vi "Defaults.vi"(8 "error in (no error)":errorcluster, 11 "MB Slave in":refnum<class "Battery Pack.lvclass">) -> (0 "error out":errorcluster, 3 "MB Slave out":refnum<class "Battery Pack.lvclass">)   [LabVIEW 2021, in "Battery Pack.lvclass"]
uses:
  Battery Pack.lvclass
  C:/Program Files (x86)/National Instruments/LabVIEW 2021/user.lib/S2 Labs/Module Framework/Modules/Base/Module.lvclass
  C:/Program Files (x86)/National Instruments/LabVIEW 2021/user.lib/S2 Labs/Module Framework/Modules/Modbus/Modbus Slave Base/Modbus Slave Base.lvclass
  <userlib>/S2 Labs/Modbus Toolkit/TypeDefs/MB Element.ctl
  <userlib>/S2 Labs/Modbus Toolkit/TypeDefs/Endianness Type.ctl
  <userlib>/S2 Labs/Modbus Toolkit/TypeDefs/Access Type.ctl
  <userlib>/S2 Labs/Module Framework/Modules/Base/Module.lvclass/Module.ctl
  <userlib>/S2 Labs/Module Framework/Modules/Modbus/Modbus Slave Base/Modbus Slave Base.lvclass/Modbus Slave Base.ctl
  <userlib>/S2 Labs/Module Framework/Modules/Base/Read Name.vi
  <userlib>/S2 Labs/Module Framework/Modules/Modbus/Modbus Slave Base/Write MB Map.vi
  <userlib>/S2 Labs/Module Framework/Modules/Base/Write Timeout (ms).vi
  MB Slave Simulator Base/MB Slave Simulator Base.lvclass
  <userlib>/S2 Labs/Modbus Toolkit/S2L Modbus API.lvclass
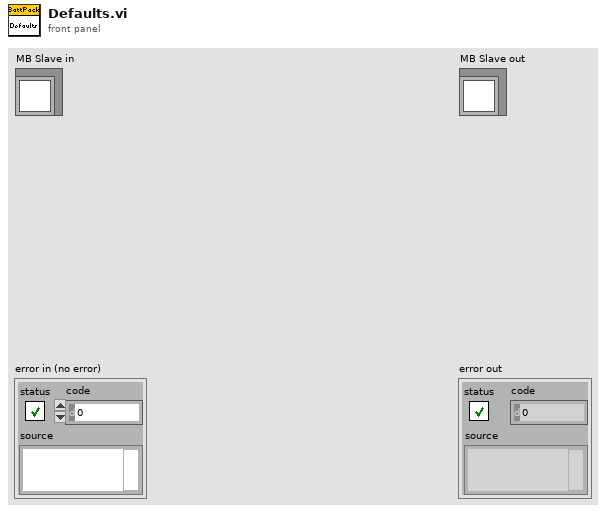
[diagram p1: front panel]
types:
  T1 = typedef "S2L Modbus API.lvclass/MB Element.ctl" = cluster{"Label":string, "Prefix":u8, "Address":u16, "Datatype":string, "Register Count":u8, "Multiplier":dbl, "Offset":dbl, "Unit":string, "Endianness":T2, "Access":T3, "LUT":string[], "Poll Rate(ms)":u16, "Mapping":cluster{"Module":string, "Channel":string}}
  T2 = typedef "Endianness Type.ctl" = enum16{"Big-Endian", "Little-Endian", "Big-Endian Byte Swap", "Little-Endian Byte Swap"}
  T3 = typedef "S2L Modbus API.lvclass/Access Type.ctl" = enum16{"R/W", "R", "W"}
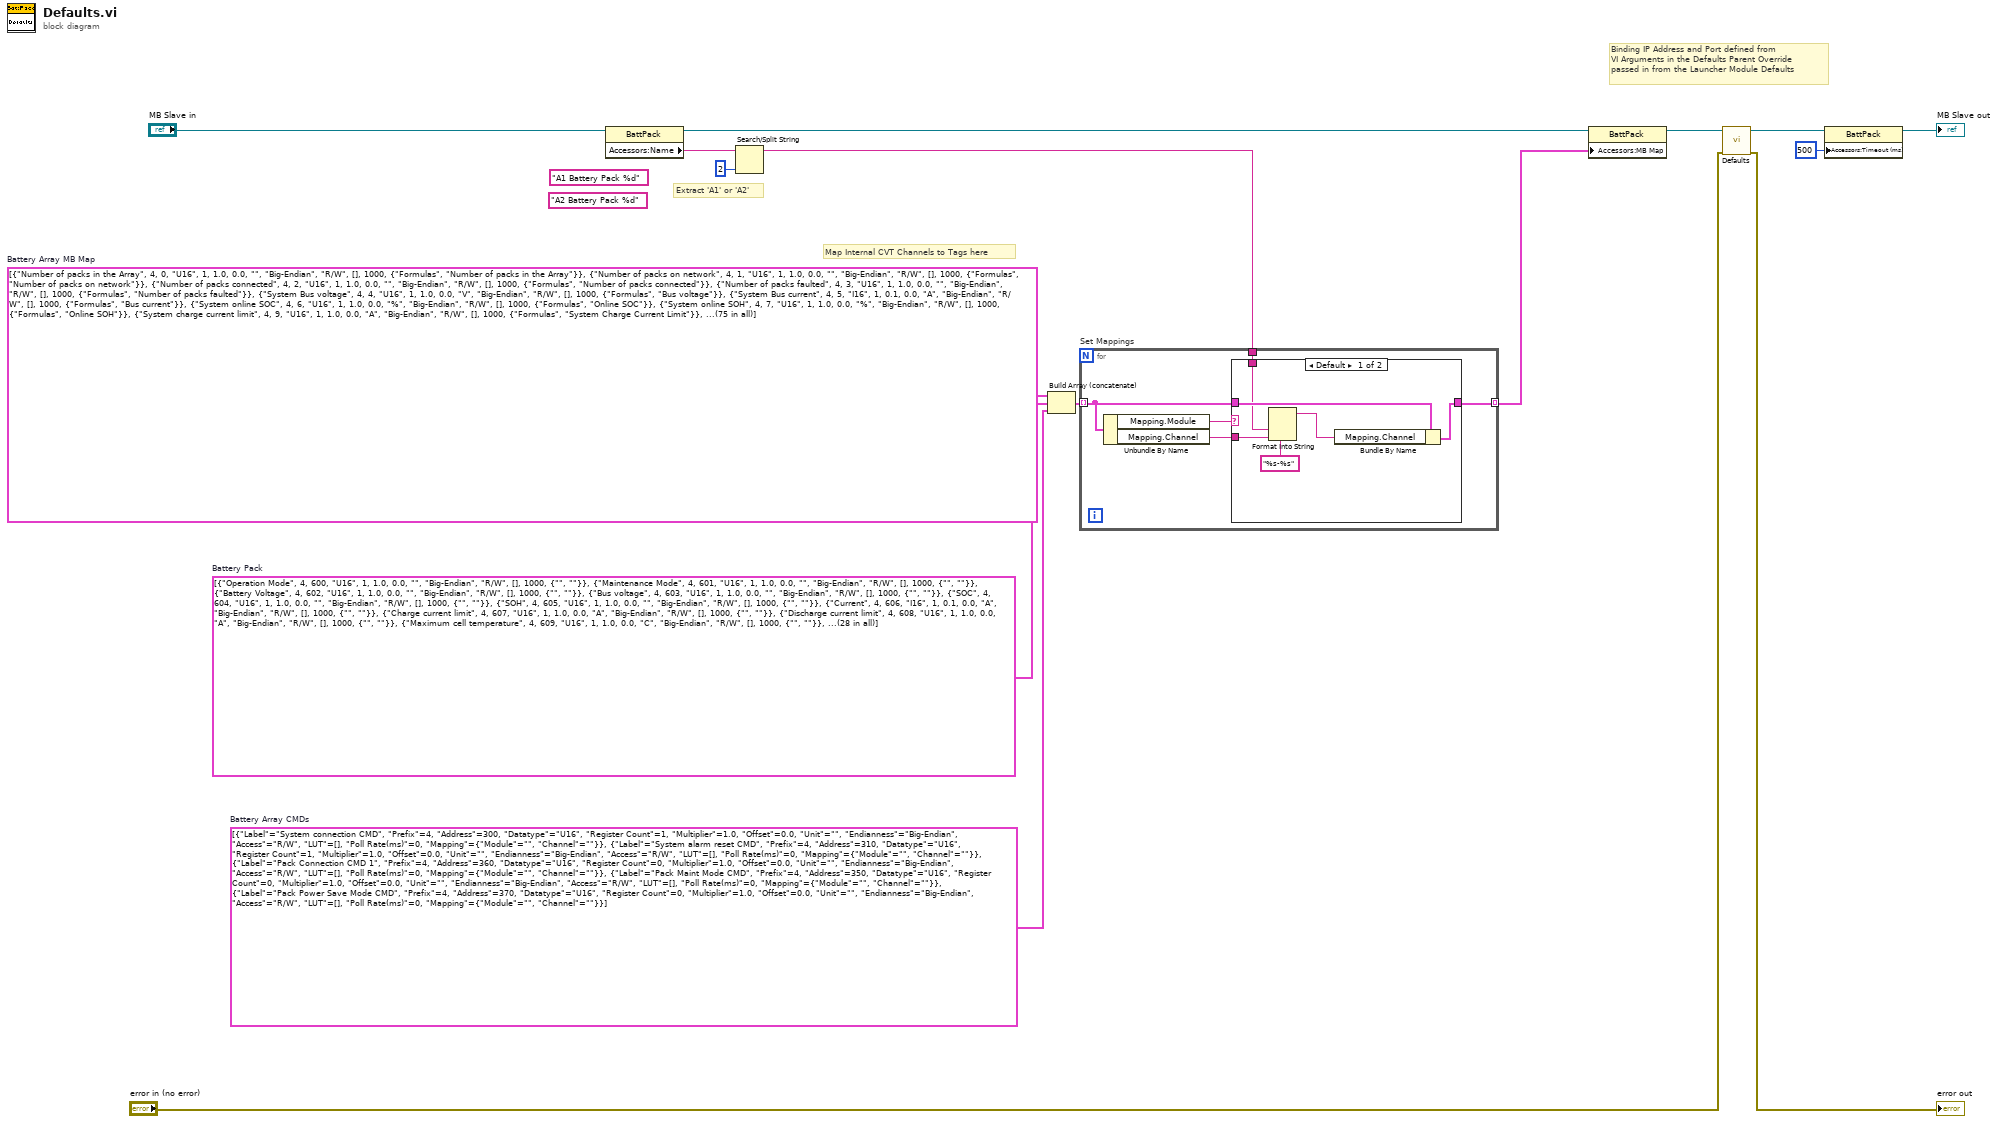
[diagram p0: block diagram]
diagram:
  (unwired) "A2 Battery Pack %d"
  (unwired) "A1 Battery Pack %d"
  w11 = T1[] [{"Label"="System connection CMD", "Prefix"=4, "Address"=300, "Datatype"="U16", "Register Count"=1, "Multiplier"=1.0, "Offset"=0.0, "Unit"="", "Endianness"=enum."Big-Endian", "Access"=enum."R/W", "LUT"=[], "Poll Rate(ms)"=0, "Mapping"={"Module"="", "Channel"=""}}, {"Label"="System alarm reset CMD", "Prefix"=4, "Address"=310, "Datatype"="U16", "Register Count"=1, "Multiplier"=1.0, "Offset"=0.0, "Unit"="", "Endianness"=enum."Big-Endian", "Access"=enum."R/W", "LUT"=[], "Poll Rate(ms)"=0, "Mapping"={"Module"="", "Channel"=""}}, {"Label"="Pack Connection CMD 1", "Prefix"=4, "Address"=360, "Datatype"="U16", "Register Count"=0, "Multiplier"=1.0, "Offset"=0.0, "Unit"="", "Endianness"=enum."Big-Endian", "Access"=enum."R/W", "LUT"=[], "Poll Rate(ms)"=0, "Mapping"={"Module"="", "Channel"=""}}, {"Label"="Pack Maint Mode CMD", "Prefix"=4, "Address"=350, "Datatype"="U16", "Register Count"=0, "Multiplier"=1.0, "Offset"=0.0, "Unit"="", "Endianness"=enum."Big-Endian", "Access"=enum."R/W", "LUT"=[], "Poll Rate(ms)"=0, "Mapping"={"Module"="", "Channel"=""}}, {"Label"="Pack Power Save Mode CMD", "Prefix"=4, "Address"=370, "Datatype"="U16", "Register Count"=0, "Multiplier"=1.0, "Offset"=0.0, "Unit"="", "Endianness"=enum."Big-Endian", "Access"=enum."R/W", "LUT"=[], "Poll Rate(ms)"=0, "Mapping"={"Module"="", "Channel"=""}}]  # Battery Array CMDs
  w13 = T1[] [{"Label"="Number of packs in the Array", "Prefix"=4, "Address"=0, "Datatype"="U16", "Register Count"=1, "Multiplier"=1.0, "Offset"=0.0, "Unit"="", "Endianness"=enum."Big-Endian", "Access"=enum."R/W", "LUT"=[], "Poll Rate(ms)"=1000, "Mapping"={"Module"="Formulas", "Channel"="Number of packs in the Array"}}, {"Label"="Number of packs on network", "Prefix"=4, "Address"=1, "Datatype"="U16", "Register Count"=1, "Multiplier"=1.0, "Offset"=0.0, "Unit"="", "Endianness"=enum."Big-Endian", "Access"=enum."R/W", "LUT"=[], "Poll Rate(ms)"=1000, "Mapping"={"Module"="Formulas", "Channel"="Number of packs on network"}}, {"Label"="Number of packs connected", "Prefix"=4, "Address"=2, "Datatype"="U16", "Register Count"=1, "Multiplier"=1.0, "Offset"=0.0, "Unit"="", "Endianness"=enum."Big-Endian", "Access"=enum."R/W", "LUT"=[], "Poll Rate(ms)"=1000, "Mapping"={"Module"="Formulas", "Channel"="Number of packs connected"}}, {"Label"="Number of packs faulted", "Prefix"=4, "Address"=3, "Datatype"="U16", "Register Count"=1, "Multiplier"=1.0, "Offset"=0.0, "Unit"="", "Endianness"=enum."Big-Endian", "Access"=enum."R/W", "LUT"=[], "Poll Rate(ms)"=1000, "Mapping"={"Module"="Formulas", "Channel"="Number of packs faulted"}}, {"Label"="System Bus voltage", "Prefix"=4, "Address"=4, "Datatype"="U16", "Register Count"=1, "Multiplier"=1.0, "Offset"=0.0, "Unit"="V", "Endianness"=enum."Big-Endian", "Access"=enum."R/W", "LUT"=[], "Poll Rate(ms)"=1000, "Mapping"={"Module"="Formulas", "Channel"="Bus voltage"}}, {"Label"="System Bus current", "Prefix"=4, "Address"=5, "Datatype"="I16", "Register Count"=1, "Multiplier"=0.1, "Offset"=0.0, "Unit"="A", "Endianness"=enum."Big-Endian", "Access"=enum."R/W", "LUT"=[], "Poll Rate(ms)"=1000, "Mapping"={"Module"="Formulas", "Channel"="Bus current"}}, {"Label"="System online SOC", "Prefix"=4, "Address"=6, "Datatype"="U16", "Register Count"=1, "Multiplier"=1.0, "Offset"=0.0, "Unit"="%", "Endianness"=enum."Big-Endian", "Access"=enum."R/W", "LUT"=[], "Poll Rate(ms)"=1000, "Mapping"={"Module"="Formulas", "Channel"="Online SOC"}}, {"Label"="System online SOH", "Prefix"=4, "Address"=7, "Datatype"="U16", "Register Count"=1, "Multiplier"=1.0, "Offset"=0.0, "Unit"="%", "Endianness"=enum."Big-Endian", "Access"=enum."R/W", "LUT"=[], "Poll Rate(ms)"=1000, "Mapping"={"Module"="Formulas", "Channel"="Online SOH"}}, {"Label"="System charge current limit", "Prefix"=4, "Address"=9, "Datatype"="U16", "Register Count"=1, "Multiplier"=1.0, "Offset"=0.0, "Unit"="A", "Endianness"=enum."Big-Endian", "Access"=enum."R/W", "LUT"=[], "Poll Rate(ms)"=1000, "Mapping"={"Module"="Formulas", "Channel"="System Charge Current Limit"}}, {"Label"="System discharge current limit", "Prefix"=4, "Address"=10, "Datatype"="U16", "Register Count"=1, "Multiplier"=1.0, "Offset"=0.0, "Unit"="A", "Endianness"=enum."Big-Endian", "Access"=enum."R/W", "LUT"=[], "Poll Rate(ms)"=1000, "Mapping"={"Module"="Formulas", "Channel"="System Discharge Current Limit"}}, {"Label"="System Maximum cell temperature", "Prefix"=4, "Address"=11, "Datatype"="I16", "Register Count"=1, "Multiplier"=1.0, "Offset"=0.0, "Unit"="C", "Endianness"=enum."Big-Endian", "Access"=enum."R/W", "LUT"=[], "Poll Rate(ms)"=1000, "Mapping"={"Module"="Formulas", "Channel"="Max Online Cell Temp"}}, {"Label"="System Minimum cell temperature", "Prefix"=4, "Address"=12, "Datatype"="I16", "Register Count"=1, "Multiplier"=1.0, "Offset"=0.0, "Unit"="C", "Endianness"=enum."Big-Endian", "Access"=enum."R/W", "LUT"=[], "Poll Rate(ms)"=1000, "Mapping"={"Module"="", "Channel"=""}}, {"Label"="System Maximum cell voltage", "Prefix"=4, "Address"=13, "Datatype"="U16", "Register Count"=1, "Multiplier"=1.0, "Offset"=0.0, "Unit"="mV", "Endianness"=enum."Big-Endian", "Access"=enum."R/W", "LUT"=[], "Poll Rate(ms)"=1000, "Mapping"={"Module"="", "Channel"=""}}, {"Label"="System Minimum cell voltage", "Prefix"=4, "Address"=14, "Datatype"="U16", "Register Count"=1, "Multiplier"=1.0, "Offset"=0.0, "Unit"="mV", "Endianness"=enum."Big-Endian", "Access"=enum."R/W", "LUT"=[], "Poll Rate(ms)"=1000, "Mapping"={"Module"="", "Channel"=""}}, {"Label"="System Maximum unconnected pack voltage", "Prefix"=4, "Address"=15, "Datatype"="U16", "Register Count"=1, "Multiplier"=1.0, "Offset"=0.0, "Unit"="V", "Endianness"=enum."Big-Endian", "Access"=enum."R/W", "LUT"=[], "Poll Rate(ms)"=1000, "Mapping"={"Module"="", "Channel"=""}}, {"Label"="System Minimum unconnected pack voltage", "Prefix"=4, "Address"=16, "Datatype"="U16", "Register Count"=1, "Multiplier"=1.0, "Offset"=0.0, "Unit"="V", "Endianness"=enum."Big-Endian", "Access"=enum."R/W", "LUT"=[], "Poll Rate(ms)"=1000, "Mapping"={"Module"="", "Channel"=""}}, {"Label"="Pack heartbeat", "Prefix"=4, "Address"=17, "Datatype"="U32", "Register Count"=1, "Multiplier"=1.0, "Offset"=0.0, "Unit"="", "Endianness"=enum."Little-Endian", "Access"=enum."R/W", "LUT"=[], "Poll Rate(ms)"=1000, "Mapping"={"Module"="", "Channel"=""}}, {"Label"="Service state", "Prefix"=4, "Address"=19, "Datatype"="U16", "Register Count"=1, "Multiplier"=1.0, "Offset"=0.0, "Unit"="", "Endianness"=enum."Big-Endian", "Access"=enum."R/W", "LUT"=[], "Poll Rate(ms)"=1000, "Mapping"={"Module"="", "Channel"=""}}, {"Label"="Bus current unscaled", "Prefix"=4, "Address"=20, "Datatype"="I16", "Register Count"=1, "Multiplier"=1.0, "Offset"=0.0, "Unit"="A", "Endianness"=enum."Big-Endian", "Access"=enum."R/W", "LUT"=[], "Poll Rate(ms)"=1000, "Mapping"={"Module"="", "Channel"=""}}, {"Label"="Minimum pack SOC", "Prefix"=4, "Address"=21, "Datatype"="U16", "Register Count"=1, "Multiplier"=1.0, "Offset"=0.0, "Unit"="%", "Endianness"=enum."Big-Endian", "Access"=enum."R/W", "LUT"=[], "Poll Rate(ms)"=0, "Mapping"={"Module"="", "Channel"=""}}, {"Label"="Average pack SOC", "Prefix"=4, "Address"=22, "Datatype"="U16", "Register Count"=1, "Multiplier"=1.0, "Offset"=0.0, "Unit"="%", "Endianness"=enum."Big-Endian", "Access"=enum."R/W", "LUT"=[], "Poll Rate(ms)"=0, "Mapping"={"Module"="", "Channel"=""}}, {"Label"="Maximum pack SOC", "Prefix"=4, "Address"=23, "Datatype"="U16", "Register Count"=1, "Multiplier"=1.0, "Offset"=0.0, "Unit"="%", "Endianness"=enum."Big-Endian", "Access"=enum."R/W", "LUT"=[], "Poll Rate(ms)"=0, "Mapping"={"Module"="", "Channel"=""}}, {"Label"="Average connected cell SOC", "Prefix"=4, "Address"=24, "Datatype"="U16", "Register Count"=1, "Multiplier"=1.0, "Offset"=0.0, "Unit"="%", "Endianness"=enum."Big-Endian", "Access"=enum."R/W", "LUT"=[], "Poll Rate(ms)"=0, "Mapping"={"Module"="", "Channel"=""}}, {"Label"="Maximum connected cell SOC", "Prefix"=4, "Address"=25, "Datatype"="U16", "Register Count"=1, "Multiplier"=1.0, "Offset"=0.0, "Unit"="%", "Endianness"=enum."Big-Endian", "Access"=enum."R/W", "LUT"=[], "Poll Rate(ms)"=0, "Mapping"={"Module"="", "Channel"=""}}, {"Label"="Pack 1 operation mode", "Prefix"=4, "Address"=50, "Datatype"="U16", "Register Count"=1, "Multiplier"=1.0, "Offset"=0.0, "Unit"="", "Endianness"=enum."Big-Endian", "Access"=enum."R/W", "LUT"=[], "Poll Rate(ms)"=1000, "Mapping"={"Module"="Formulas", "Channel"="Pack 1 operation mode"}}, {"Label"="Pack 2 operation mode", "Prefix"=4, "Address"=51, "Datatype"="U16", "Register Count"=1, "Multiplier"=1.0, "Offset"=0.0, "Unit"="", "Endianness"=enum."Big-Endian", "Access"=enum."R/W", "LUT"=[], "Poll Rate(ms)"=1000, "Mapping"={"Module"="Formulas", "Channel"="Pack 2 operation mode"}}, {"Label"="Pack 3 operation mode", "Prefix"=4, "Address"=52, "Datatype"="U16", "Register Count"=1, "Multiplier"=1.0, "Offset"=0.0, "Unit"="", "Endianness"=enum."Big-Endian", "Access"=enum."R/W", "LUT"=[], "Poll Rate(ms)"=1000, "Mapping"={"Module"="Formulas", "Channel"="Pack 3 operation mode"}}, {"Label"="Pack 4 operation mode", "Prefix"=4, "Address"=53, "Datatype"="U16", "Register Count"=1, "Multiplier"=1.0, "Offset"=0.0, "Unit"="", "Endianness"=enum."Big-Endian", "Access"=enum."R/W", "LUT"=[], "Poll Rate(ms)"=1000, "Mapping"={"Module"="Formulas", "Channel"="Pack 4 operation mode"}}, {"Label"="Pack 5 operation mode", "Prefix"=4, "Address"=54, "Datatype"="U16", "Register Count"=1, "Multiplier"=1.0, "Offset"=0.0, "Unit"="", "Endianness"=enum."Big-Endian", "Access"=enum."R/W", "LUT"=[], "Poll Rate(ms)"=1000, "Mapping"={"Module"="Formulas", "Channel"="Pack 5 operation mode"}}, {"Label"="Pack 6 operation mode", "Prefix"=4, "Address"=55, "Datatype"="U16", "Register Count"=1, "Multiplier"=1.0, "Offset"=0.0, "Unit"="", "Endianness"=enum."Big-Endian", "Access"=enum."R/W", "LUT"=[], "Poll Rate(ms)"=1000, "Mapping"={"Module"="Formulas", "Channel"="Pack 6 operation mode"}}, {"Label"="Pack 1 maintenance status", "Prefix"=4, "Address"=66, "Datatype"="U16", "Register Count"=1, "Multiplier"=1.0, "Offset"=0.0, "Unit"="", "Endianness"=enum."Big-Endian", "Access"=enum."R/W", "LUT"=[], "Poll Rate(ms)"=1000, "Mapping"={"Module"="", "Channel"=""}}, {"Label"="Pack 2 maintenance status", "Prefix"=4, "Address"=67, "Datatype"="U16", "Register Count"=1, "Multiplier"=1.0, "Offset"=0.0, "Unit"="", "Endianness"=enum."Big-Endian", "Access"=enum."R/W", "LUT"=[], "Poll Rate(ms)"=1000, "Mapping"={"Module"="", "Channel"=""}}, {"Label"="Pack 3 maintenance status", "Prefix"=4, "Address"=68, "Datatype"="U16", "Register Count"=1, "Multiplier"=1.0, "Offset"=0.0, "Unit"="", "Endianness"=enum."Big-Endian", "Access"=enum."R/W", "LUT"=[], "Poll Rate(ms)"=1000, "Mapping"={"Module"="", "Channel"=""}}, {"Label"="Pack 4 maintenance status", "Prefix"=4, "Address"=69, "Datatype"="U16", "Register Count"=1, "Multiplier"=1.0, "Offset"=0.0, "Unit"="", "Endianness"=enum."Big-Endian", "Access"=enum."R/W", "LUT"=[], "Poll Rate(ms)"=1000, "Mapping"={"Module"="", "Channel"=""}}, {"Label"="Pack 5 maintenance status", "Prefix"=4, "Address"=70, "Datatype"="U16", "Register Count"=1, "Multiplier"=1.0, "Offset"=0.0, "Unit"="", "Endianness"=enum."Big-Endian", "Access"=enum."R/W", "LUT"=[], "Poll Rate(ms)"=1000, "Mapping"={"Module"="", "Channel"=""}}, {"Label"="Pack 6 maintenance status", "Prefix"=4, "Address"=71, "Datatype"="U16", "Register Count"=1, "Multiplier"=1.0, "Offset"=0.0, "Unit"="", "Endianness"=enum."Big-Endian", "Access"=enum."R/W", "LUT"=[], "Poll Rate(ms)"=1000, "Mapping"={"Module"="", "Channel"=""}}, {"Label"="Pack 1 pre-charge status", "Prefix"=4, "Address"=82, "Datatype"="U16", "Register Count"=1, "Multiplier"=1.0, "Offset"=0.0, "Unit"="", "Endianness"=enum."Big-Endian", "Access"=enum."R/W", "LUT"=[], "Poll Rate(ms)"=1000, "Mapping"={"Module"="", "Channel"=""}}, {"Label"="Pack 2 pre-charge status", "Prefix"=4, "Address"=83, "Datatype"="U16", "Register Count"=1, "Multiplier"=1.0, "Offset"=0.0, "Unit"="", "Endianness"=enum."Big-Endian", "Access"=enum."R/W", "LUT"=[], "Poll Rate(ms)"=1000, "Mapping"={"Module"="", "Channel"=""}}, {"Label"="Pack 3 pre-charge status", "Prefix"=4, "Address"=84, "Datatype"="U16", "Register Count"=1, "Multiplier"=1.0, "Offset"=0.0, "Unit"="", "Endianness"=enum."Big-Endian", "Access"=enum."R/W", "LUT"=[], "Poll Rate(ms)"=1000, "Mapping"={"Module"="", "Channel"=""}}, {"Label"="Pack 4 pre-charge status", "Prefix"=4, "Address"=85, "Datatype"="U16", "Register Count"=1, "Multiplier"=1.0, "Offset"=0.0, "Unit"="", "Endianness"=enum."Big-Endian", "Access"=enum."R/W", "LUT"=[], "Poll Rate(ms)"=1000, "Mapping"={"Module"="", "Channel"=""}}, {"Label"="Pack 5 pre-charge status", "Prefix"=4, "Address"=86, "Datatype"="U16", "Register Count"=1, "Multiplier"=1.0, "Offset"=0.0, "Unit"="", "Endianness"=enum."Big-Endian", "Access"=enum."R/W", "LUT"=[], "Poll Rate(ms)"=1000, "Mapping"={"Module"="", "Channel"=""}}, {"Label"="Pack 6 pre-charge status", "Prefix"=4, "Address"=87, "Datatype"="U16", "Register Count"=1, "Multiplier"=1.0, "Offset"=0.0, "Unit"="", "Endianness"=enum."Big-Endian", "Access"=enum."R/W", "LUT"=[], "Poll Rate(ms)"=1000, "Mapping"={"Module"="", "Channel"=""}}, {"Label"="Pack 1 connection feedback", "Prefix"=4, "Address"=98, "Datatype"="U16", "Register Count"=1, "Multiplier"=1.0, "Offset"=0.0, "Unit"="", "Endianness"=enum."Big-Endian", "Access"=enum."R/W", "LUT"=[], "Poll Rate(ms)"=1000, "Mapping"={"Module"="", "Channel"=""}}, {"Label"="Pack 2 connection feedback", "Prefix"=4, "Address"=99, "Datatype"="U16", "Register Count"=1, "Multiplier"=1.0, "Offset"=0.0, "Unit"="", "Endianness"=enum."Big-Endian", "Access"=enum."R/W", "LUT"=[], "Poll Rate(ms)"=1000, "Mapping"={"Module"="", "Channel"=""}}, {"Label"="Pack 3 connection feedback", "Prefix"=4, "Address"=100, "Datatype"="U16", "Register Count"=1, "Multiplier"=1.0, "Offset"=0.0, "Unit"="", "Endianness"=enum."Big-Endian", "Access"=enum."R/W", "LUT"=[], "Poll Rate(ms)"=1000, "Mapping"={"Module"="", "Channel"=""}}, {"Label"="Pack 4 connection feedback", "Prefix"=4, "Address"=101, "Datatype"="U16", "Register Count"=1, "Multiplier"=1.0, "Offset"=0.0, "Unit"="", "Endianness"=enum."Big-Endian", "Access"=enum."R/W", "LUT"=[], "Poll Rate(ms)"=1000, "Mapping"={"Module"="", "Channel"=""}}, {"Label"="Pack 5 connection feedback", "Prefix"=4, "Address"=102, "Datatype"="U16", "Register Count"=1, "Multiplier"=1.0, "Offset"=0.0, "Unit"="", "Endianness"=enum."Big-Endian", "Access"=enum."R/W", "LUT"=[], "Poll Rate(ms)"=1000, "Mapping"={"Module"="", "Channel"=""}}, {"Label"="Pack 6 connection feedback", "Prefix"=4, "Address"=103, "Datatype"="U16", "Register Count"=1, "Multiplier"=1.0, "Offset"=0.0, "Unit"="", "Endianness"=enum."Big-Endian", "Access"=enum."R/W", "LUT"=[], "Poll Rate(ms)"=1000, "Mapping"={"Module"="", "Channel"=""}}, {"Label"="Pack 1 pre-charge bypass feedback", "Prefix"=4, "Address"=114, "Datatype"="U16", "Register Count"=1, "Multiplier"=1.0, "Offset"=0.0, "Unit"="", "Endianness"=enum."Big-Endian", "Access"=enum."R/W", "LUT"=[], "Poll Rate(ms)"=1000, "Mapping"={"Module"="", "Channel"=""}}, {"Label"="Pack 2 pre-charge bypass feedback", "Prefix"=4, "Address"=115, "Datatype"="U16", "Register Count"=1, "Multiplier"=1.0, "Offset"=0.0, "Unit"="", "Endianness"=enum."Big-Endian", "Access"=enum."R/W", "LUT"=[], "Poll Rate(ms)"=1000, "Mapping"={"Module"="", "Channel"=""}}, {"Label"="Pack 3 pre-charge bypass feedback", "Prefix"=4, "Address"=116, "Datatype"="U16", "Register Count"=1, "Multiplier"=1.0, "Offset"=0.0, "Unit"="", "Endianness"=enum."Big-Endian", "Access"=enum."R/W", "LUT"=[], "Poll Rate(ms)"=1000, "Mapping"={"Module"="", "Channel"=""}}, {"Label"="Pack 4 pre-charge bypass feedback", "Prefix"=4, "Address"=117, "Datatype"="U16", "Register Count"=1, "Multiplier"=1.0, "Offset"=0.0, "Unit"="", "Endianness"=enum."Big-Endian", "Access"=enum."R/W", "LUT"=[], "Poll Rate(ms)"=1000, "Mapping"={"Module"="", "Channel"=""}}, {"Label"="Pack 5 pre-charge bypass feedback", "Prefix"=4, "Address"=118, "Datatype"="U16", "Register Count"=1, "Multiplier"=1.0, "Offset"=0.0, "Unit"="", "Endianness"=enum."Big-Endian", "Access"=enum."R/W", "LUT"=[], "Poll Rate(ms)"=1000, "Mapping"={"Module"="", "Channel"=""}}, {"Label"="Pack 6 pre-charge bypass feedback", "Prefix"=4, "Address"=119, "Datatype"="U16", "Register Count"=1, "Multiplier"=1.0, "Offset"=0.0, "Unit"="", "Endianness"=enum."Big-Endian", "Access"=enum."R/W", "LUT"=[], "Poll Rate(ms)"=1000, "Mapping"={"Module"="", "Channel"=""}}, {"Label"="Pack 1 alarm status", "Prefix"=4, "Address"=400, "Datatype"="Bit Flag", "Register Count"=1, "Multiplier"=1.0, "Offset"=0.0, "Unit"="", "Endianness"=enum."Big-Endian", "Access"=enum."R/W", "LUT"=["Fault", "Warning"], "Poll Rate(ms)"=1000, "Mapping"={"Module"="", "Channel"=""}}, {"Label"="Pack 1 fault status", "Prefix"=4, "Address"=401, "Datatype"="Bit Flag", "Register Count"=1, "Multiplier"=1.0, "Offset"=0.0, "Unit"="", "Endianness"=enum."Big-Endian", "Access"=enum."R/W", "LUT"=["SE over voltage fault", "SE under voltage fault", "SE over temperature fault", "HVIL fault", "E-stop active fault", "Safety shutdown fault", "Pack ground fault", "Contactor fail fault", "Low temperature overcurrent fault"], "Poll Rate(ms)"=1000, "Mapping"={"Module"="", "Channel"=""}}, {"Label"="Pack 1 warning status", "Prefix"=4, "Address"=403, "Datatype"="Bit Flag", "Register Count"=1, "Multiplier"=1.0, "Offset"=0.0, "Unit"="", "Endianness"=enum."Big-Endian", "Access"=enum."R/W", "LUT"=["SE over voltage warning", "SE under voltage warning", "SE over temperature warning", "Communication warning", "Over current warning", "Input power loss warning", "PDM over temperature warning", "Reserved", "Fuse failure warning"], "Poll Rate(ms)"=1000, "Mapping"={"Module"="", "Channel"=""}}, {"Label"="Pack 2 alarm status", "Prefix"=4, "Address"=405, "Datatype"="Bit Flag", "Register Count"=1, "Multiplier"=1.0, "Offset"=0.0, "Unit"="", "Endianness"=enum."Big-Endian", "Access"=enum."R/W", "LUT"=["Fault", "Warning"], "Poll Rate(ms)"=1000, "Mapping"={"Module"="", "Channel"=""}}, {"Label"="Pack 2 fault status", "Prefix"=4, "Address"=406, "Datatype"="Bit Flag", "Register Count"=1, "Multiplier"=1.0, "Offset"=0.0, "Unit"="", "Endianness"=enum."Big-Endian", "Access"=enum."R/W", "LUT"=["SE over voltage fault", "SE under voltage fault", "SE over temperature fault", "HVIL fault", "E-stop active fault", "Safety shutdown fault", "Pack ground fault", "Contactor fail fault", "Low temperature overcurrent fault"], "Poll Rate(ms)"=1000, "Mapping"={"Module"="", "Channel"=""}}, {"Label"="Pack 2 warning status", "Prefix"=4, "Address"=408, "Datatype"="Bit Flag", "Register Count"=1, "Multiplier"=1.0, "Offset"=0.0, "Unit"="", "Endianness"=enum."Big-Endian", "Access"=enum."R/W", "LUT"=["SE over voltage warning", "SE under voltage warning", "SE over temperature warning", "Communication warning", "Over current warning", "Input power loss warning", "PDM over temperature warning", "Reserved", "Fuse failure warning"], "Poll Rate(ms)"=1000, "Mapping"={"Module"="", "Channel"=""}}, {"Label"="Pack 3 alarm status", "Prefix"=4, "Address"=410, "Datatype"="Bit Flag", "Register Count"=1, "Multiplier"=1.0, "Offset"=0.0, "Unit"="", "Endianness"=enum."Big-Endian", "Access"=enum."R/W", "LUT"=["Fault", "Warning"], "Poll Rate(ms)"=1000, "Mapping"={"Module"="", "Channel"=""}}, {"Label"="Pack 3 fault status", "Prefix"=4, "Address"=411, "Datatype"="Bit Flag", "Register Count"=1, "Multiplier"=1.0, "Offset"=0.0, "Unit"="", "Endianness"=enum."Big-Endian", "Access"=enum."R/W", "LUT"=["SE over voltage fault", "SE under voltage fault", "SE over temperature fault", "HVIL fault", "E-stop active fault", "Safety shutdown fault", "Pack ground fault", "Contactor fail fault", "Low temperature overcurrent fault"], "Poll Rate(ms)"=1000, "Mapping"={"Module"="", "Channel"=""}}, {"Label"="Pack 3 warning status", "Prefix"=4, "Address"=413, "Datatype"="Bit Flag", "Register Count"=1, "Multiplier"=1.0, "Offset"=0.0, "Unit"="", "Endianness"=enum."Big-Endian", "Access"=enum."R/W", "LUT"=["SE over voltage warning", "SE under voltage warning", "SE over temperature warning", "Communication warning", "Over current warning", "Input power loss warning", "PDM over temperature warning", "Reserved", "Fuse failure warning"], "Poll Rate(ms)"=1000, "Mapping"={"Module"="", "Channel"=""}}, {"Label"="Pack 4 alarm status", "Prefix"=4, "Address"=415, "Datatype"="Bit Flag", "Register Count"=1, "Multiplier"=1.0, "Offset"=0.0, "Unit"="", "Endianness"=enum."Big-Endian", "Access"=enum."R/W", "LUT"=["Fault", "Warning"], "Poll Rate(ms)"=1000, "Mapping"={"Module"="", "Channel"=""}}, {"Label"="Pack 4 fault status", "Prefix"=4, "Address"=416, "Datatype"="Bit Flag", "Register Count"=1, "Multiplier"=1.0, "Offset"=0.0, "Unit"="", "Endianness"=enum."Big-Endian", "Access"=enum."R/W", "LUT"=["SE over voltage fault", "SE under voltage fault", "SE over temperature fault", "HVIL fault", "E-stop active fault", "Safety shutdown fault", "Pack ground fault", "Contactor fail fault", "Low temperature overcurrent fault"], "Poll Rate(ms)"=1000, "Mapping"={"Module"="", "Channel"=""}}, {"Label"="Pack 4 warning status", "Prefix"=4, "Address"=418, "Datatype"="Bit Flag", "Register Count"=1, "Multiplier"=1.0, "Offset"=0.0, "Unit"="", "Endianness"=enum."Big-Endian", "Access"=enum."R/W", "LUT"=["SE over voltage warning", "SE under voltage warning", "SE over temperature warning", "Communication warning", "Over current warning", "Input power loss warning", "PDM over temperature warning", "Reserved", "Fuse failure warning"], "Poll Rate(ms)"=1000, "Mapping"={"Module"="", "Channel"=""}}, {"Label"="Pack 5 alarm status", "Prefix"=4, "Address"=420, "Datatype"="Bit Flag", "Register Count"=1, "Multiplier"=1.0, "Offset"=0.0, "Unit"="", "Endianness"=enum."Big-Endian", "Access"=enum."R/W", "LUT"=["Fault", "Warning"], "Poll Rate(ms)"=1000, "Mapping"={"Module"="", "Channel"=""}}, {"Label"="Pack 5 fault status", "Prefix"=4, "Address"=421, "Datatype"="Bit Flag", "Register Count"=1, "Multiplier"=1.0, "Offset"=0.0, "Unit"="", "Endianness"=enum."Big-Endian", "Access"=enum."R/W", "LUT"=["SE over voltage fault", "SE under voltage fault", "SE over temperature fault", "HVIL fault", "E-stop active fault", "Safety shutdown fault", "Pack ground fault", "Contactor fail fault", "Low temperature overcurrent fault"], "Poll Rate(ms)"=1000, "Mapping"={"Module"="", "Channel"=""}}, {"Label"="Pack 5 warning status", "Prefix"=4, "Address"=423, "Datatype"="Bit Flag", "Register Count"=1, "Multiplier"=1.0, "Offset"=0.0, "Unit"="", "Endianness"=enum."Big-Endian", "Access"=enum."R/W", "LUT"=["SE over voltage warning", "SE under voltage warning", "SE over temperature warning", "Communication warning", "Over current warning", "Input power loss warning", "PDM over temperature warning", "Reserved", "Fuse failure warning"], "Poll Rate(ms)"=1000, "Mapping"={"Module"="", "Channel"=""}}, {"Label"="Pack 6 alarm status", "Prefix"=4, "Address"=425, "Datatype"="Bit Flag", "Register Count"=1, "Multiplier"=1.0, "Offset"=0.0, "Unit"="", "Endianness"=enum."Big-Endian", "Access"=enum."R/W", "LUT"=["Fault", "Warning"], "Poll Rate(ms)"=1000, "Mapping"={"Module"="", "Channel"=""}}, {"Label"="Pack 6 fault status", "Prefix"=4, "Address"=426, "Datatype"="Bit Flag", "Register Count"=1, "Multiplier"=1.0, "Offset"=0.0, "Unit"="", "Endianness"=enum."Big-Endian", "Access"=enum."R/W", "LUT"=["SE over voltage fault", "SE under voltage fault", "SE over temperature fault", "HVIL fault", "E-stop active fault", "Safety shutdown fault", "Pack ground fault", "Contactor fail fault", "Low temperature overcurrent fault"], "Poll Rate(ms)"=1000, "Mapping"={"Module"="", "Channel"=""}}, {"Label"="Pack 6 warning status", "Prefix"=4, "Address"=427, "Datatype"="Bit Flag", "Register Count"=1, "Multiplier"=1.0, "Offset"=0.0, "Unit"="", "Endianness"=enum."Big-Endian", "Access"=enum."R/W", "LUT"=["SE over voltage warning", "SE under voltage warning", "SE over temperature warning", "Communication warning", "Over current warning", "Input power loss warning", "PDM over temperature warning", "Reserved", "Fuse failure warning"], "Poll Rate(ms)"=1000, "Mapping"={"Module"="", "Channel"=""}}, {"Label"="System connection CMD Ack", "Prefix"=4, "Address"=301, "Datatype"="U32", "Register Count"=1, "Multiplier"=1.0, "Offset"=0.0, "Unit"="", "Endianness"=enum."Little-Endian", "Access"=enum."R/W", "LUT"=[], "Poll Rate(ms)"=1000, "Mapping"={"Module"="", "Channel"=""}}, {"Label"="System alarm reset CMD Ack", "Prefix"=4, "Address"=311, "Datatype"="U32", "Register Count"=1, "Multiplier"=1.0, "Offset"=0.0, "Unit"="", "Endianness"=enum."Little-Endian", "Access"=enum."R/W", "LUT"=[], "Poll Rate(ms)"=1000, "Mapping"={"Module"="", "Channel"=""}}, {"Label"="Pack connection CMD Ack", "Prefix"=4, "Address"=362, "Datatype"="U32", "Register Count"=1, "Multiplier"=1.0, "Offset"=0.0, "Unit"="", "Endianness"=enum."Little-Endian", "Access"=enum."R/W", "LUT"=[], "Poll Rate(ms)"=1000, "Mapping"={"Module"="", "Channel"=""}}]  # Battery Array MB Map
  w12 = T1[] [{"Label"="Operation Mode", "Prefix"=4, "Address"=600, "Datatype"="U16", "Register Count"=1, "Multiplier"=1.0, "Offset"=0.0, "Unit"="", "Endianness"=enum."Big-Endian", "Access"=enum."R/W", "LUT"=[], "Poll Rate(ms)"=1000, "Mapping"={"Module"="", "Channel"=""}}, {"Label"="Maintenance Mode", "Prefix"=4, "Address"=601, "Datatype"="U16", "Register Count"=1, "Multiplier"=1.0, "Offset"=0.0, "Unit"="", "Endianness"=enum."Big-Endian", "Access"=enum."R/W", "LUT"=[], "Poll Rate(ms)"=1000, "Mapping"={"Module"="", "Channel"=""}}, {"Label"="Battery Voltage", "Prefix"=4, "Address"=602, "Datatype"="U16", "Register Count"=1, "Multiplier"=1.0, "Offset"=0.0, "Unit"="", "Endianness"=enum."Big-Endian", "Access"=enum."R/W", "LUT"=[], "Poll Rate(ms)"=1000, "Mapping"={"Module"="", "Channel"=""}}, {"Label"="Bus voltage", "Prefix"=4, "Address"=603, "Datatype"="U16", "Register Count"=1, "Multiplier"=1.0, "Offset"=0.0, "Unit"="", "Endianness"=enum."Big-Endian", "Access"=enum."R/W", "LUT"=[], "Poll Rate(ms)"=1000, "Mapping"={"Module"="", "Channel"=""}}, {"Label"="SOC", "Prefix"=4, "Address"=604, "Datatype"="U16", "Register Count"=1, "Multiplier"=1.0, "Offset"=0.0, "Unit"="", "Endianness"=enum."Big-Endian", "Access"=enum."R/W", "LUT"=[], "Poll Rate(ms)"=1000, "Mapping"={"Module"="", "Channel"=""}}, {"Label"="SOH", "Prefix"=4, "Address"=605, "Datatype"="U16", "Register Count"=1, "Multiplier"=1.0, "Offset"=0.0, "Unit"="", "Endianness"=enum."Big-Endian", "Access"=enum."R/W", "LUT"=[], "Poll Rate(ms)"=1000, "Mapping"={"Module"="", "Channel"=""}}, {"Label"="Current", "Prefix"=4, "Address"=606, "Datatype"="I16", "Register Count"=1, "Multiplier"=0.1, "Offset"=0.0, "Unit"="A", "Endianness"=enum."Big-Endian", "Access"=enum."R/W", "LUT"=[], "Poll Rate(ms)"=1000, "Mapping"={"Module"="", "Channel"=""}}, {"Label"="Charge current limit", "Prefix"=4, "Address"=607, "Datatype"="U16", "Register Count"=1, "Multiplier"=1.0, "Offset"=0.0, "Unit"="A", "Endianness"=enum."Big-Endian", "Access"=enum."R/W", "LUT"=[], "Poll Rate(ms)"=1000, "Mapping"={"Module"="", "Channel"=""}}, {"Label"="Discharge current limit", "Prefix"=4, "Address"=608, "Datatype"="U16", "Register Count"=1, "Multiplier"=1.0, "Offset"=0.0, "Unit"="A", "Endianness"=enum."Big-Endian", "Access"=enum."R/W", "LUT"=[], "Poll Rate(ms)"=1000, "Mapping"={"Module"="", "Channel"=""}}, {"Label"="Maximum cell temperature", "Prefix"=4, "Address"=609, "Datatype"="U16", "Register Count"=1, "Multiplier"=1.0, "Offset"=0.0, "Unit"="C", "Endianness"=enum."Big-Endian", "Access"=enum."R/W", "LUT"=[], "Poll Rate(ms)"=1000, "Mapping"={"Module"="", "Channel"=""}}, {"Label"="Minimum cell temperature", "Prefix"=4, "Address"=610, "Datatype"="U16", "Register Count"=1, "Multiplier"=1.0, "Offset"=0.0, "Unit"="C", "Endianness"=enum."Big-Endian", "Access"=enum."R/W", "LUT"=[], "Poll Rate(ms)"=1000, "Mapping"={"Module"="", "Channel"=""}}, {"Label"="Maximum cell voltage", "Prefix"=4, "Address"=611, "Datatype"="U16", "Register Count"=1, "Multiplier"=1.0, "Offset"=0.0, "Unit"="mV", "Endianness"=enum."Big-Endian", "Access"=enum."R/W", "LUT"=[], "Poll Rate(ms)"=1000, "Mapping"={"Module"="", "Channel"=""}}, {"Label"="Minimum cell voltage", "Prefix"=4, "Address"=612, "Datatype"="U16", "Register Count"=1, "Multiplier"=1.0, "Offset"=0.0, "Unit"="mV", "Endianness"=enum."Big-Endian", "Access"=enum."R/W", "LUT"=[], "Poll Rate(ms)"=1000, "Mapping"={"Module"="", "Channel"=""}}, {"Label"="Reserved1", "Prefix"=4, "Address"=613, "Datatype"="U16", "Register Count"=1, "Multiplier"=1.0, "Offset"=0.0, "Unit"="", "Endianness"=enum."Big-Endian", "Access"=enum."R/W", "LUT"=[], "Poll Rate(ms)"=1000, "Mapping"={"Module"="", "Channel"=""}}, {"Label"="Reserved2", "Prefix"=4, "Address"=614, "Datatype"="U16", "Register Count"=1, "Multiplier"=1.0, "Offset"=0.0, "Unit"="", "Endianness"=enum."Big-Endian", "Access"=enum."R/W", "LUT"=[], "Poll Rate(ms)"=1000, "Mapping"={"Module"="", "Channel"=""}}, {"Label"="Service required", "Prefix"=4, "Address"=615, "Datatype"="U16", "Register Count"=1, "Multiplier"=1.0, "Offset"=0.0, "Unit"="", "Endianness"=enum."Big-Endian", "Access"=enum."R/W", "LUT"=[], "Poll Rate(ms)"=1000, "Mapping"={"Module"="", "Channel"=""}}, {"Label"="Service code", "Prefix"=4, "Address"=616, "Datatype"="U64", "Register Count"=1, "Multiplier"=1.0, "Offset"=0.0, "Unit"="", "Endianness"=enum."Little-Endian", "Access"=enum."R/W", "LUT"=[], "Poll Rate(ms)"=1000, "Mapping"={"Module"="", "Channel"=""}}, {"Label"="Reserved3", "Prefix"=4, "Address"=620, "Datatype"="U16", "Register Count"=1, "Multiplier"=1.0, "Offset"=0.0, "Unit"="", "Endianness"=enum."Big-Endian", "Access"=enum."R/W", "LUT"=[], "Poll Rate(ms)"=1000, "Mapping"={"Module"="", "Channel"=""}}, {"Label"="Reserved4", "Prefix"=4, "Address"=621, "Datatype"="U16", "Register Count"=1, "Multiplier"=1.0, "Offset"=0.0, "Unit"="", "Endianness"=enum."Big-Endian", "Access"=enum."R/W", "LUT"=[], "Poll Rate(ms)"=1000, "Mapping"={"Module"="", "Channel"=""}}, {"Label"="Reserved5", "Prefix"=4, "Address"=622, "Datatype"="U16", "Register Count"=1, "Multiplier"=1.0, "Offset"=0.0, "Unit"="", "Endianness"=enum."Big-Endian", "Access"=enum."R/W", "LUT"=[], "Poll Rate(ms)"=1000, "Mapping"={"Module"="", "Channel"=""}}, {"Label"="Reserved6", "Prefix"=4, "Address"=623, "Datatype"="U16", "Register Count"=1, "Multiplier"=1.0, "Offset"=0.0, "Unit"="", "Endianness"=enum."Big-Endian", "Access"=enum."R/W", "LUT"=[], "Poll Rate(ms)"=1000, "Mapping"={"Module"="", "Channel"=""}}, {"Label"="Reserved7", "Prefix"=4, "Address"=624, "Datatype"="U16", "Register Count"=1, "Multiplier"=1.0, "Offset"=0.0, "Unit"="", "Endianness"=enum."Big-Endian", "Access"=enum."R/W", "LUT"=[], "Poll Rate(ms)"=1000, "Mapping"={"Module"="", "Channel"=""}}, {"Label"="Average cell temperature", "Prefix"=4, "Address"=625, "Datatype"="U16", "Register Count"=1, "Multiplier"=1.0, "Offset"=0.0, "Unit"="C", "Endianness"=enum."Big-Endian", "Access"=enum."R/W", "LUT"=[], "Poll Rate(ms)"=1000, "Mapping"={"Module"="", "Channel"=""}}, {"Label"="Average cell voltage", "Prefix"=4, "Address"=626, "Datatype"="U16", "Register Count"=1, "Multiplier"=1.0, "Offset"=0.0, "Unit"="mV", "Endianness"=enum."Big-Endian", "Access"=enum."R/W", "LUT"=[], "Poll Rate(ms)"=1000, "Mapping"={"Module"="", "Channel"=""}}, {"Label"="Cell balancing status", "Prefix"=4, "Address"=627, "Datatype"="U16", "Register Count"=1, "Multiplier"=1.0, "Offset"=0.0, "Unit"="", "Endianness"=enum."Big-Endian", "Access"=enum."R/W", "LUT"=[], "Poll Rate(ms)"=1000, "Mapping"={"Module"="", "Channel"=""}}, {"Label"="Cells out of balance", "Prefix"=4, "Address"=628, "Datatype"="U16", "Register Count"=1, "Multiplier"=1.0, "Offset"=0.0, "Unit"="", "Endianness"=enum."Big-Endian", "Access"=enum."R/W", "LUT"=[], "Poll Rate(ms)"=1000, "Mapping"={"Module"="", "Channel"=""}}, {"Label"="Black-start button status", "Prefix"=4, "Address"=629, "Datatype"="U16", "Register Count"=1, "Multiplier"=1.0, "Offset"=0.0, "Unit"="", "Endianness"=enum."Big-Endian", "Access"=enum."R/W", "LUT"=[], "Poll Rate(ms)"=1000, "Mapping"={"Module"="", "Channel"=""}}, {"Label"="Pre-charge resistor energy", "Prefix"=4, "Address"=630, "Datatype"="U16", "Register Count"=1, "Multiplier"=0.1, "Offset"=0.0, "Unit"="%", "Endianness"=enum."Big-Endian", "Access"=enum."R/W", "LUT"=[], "Poll Rate(ms)"=1000, "Mapping"={"Module"="", "Channel"=""}}]  # Battery Pack
  # "Extract 'A1' or 'A2'"
  # "Binding IP Address and Port defined from\nVI Arguments in the Defaults Parent Override\npassed in from the Launcher Module Defaults"
  # "Map Internal CVT Channels to Tags here"
  n1 = property class="BattPack"(reference="MB Slave in") -> (reference out=w9:refnum<class "Battery Pack.lvclass">, "Accessors:Name"=w7:string)  [unwired: 1 in, 1 out]
  n2 = Search/Split String(string=w7, offset (0)=2) -> (substring before match=w4:string)  [unwired: 1 in, 2 out]
  n3 = Build Array (concatenate)(w13, w12, w11) -> (w5:T1[])
  n4 = for "Set Mappings" {
    tunnel: [w20] -> w6 mode=indexing
    tunnel: w5 -> [w19] mode=indexing
    tunnel: w4 -> [w17]
    n5 = Unbundle By Name(w19) -> ("Mapping.Module"=w21:string, "Mapping.Channel"=w18:string)
    n6 = case shown="Default" w21 {
      tunnel: [w26 w28] -> w20
      tunnel: w19 -> [w27 w28]
      tunnel: w18 -> [w23 _]
      tunnel: w17 -> [w24 _]
      frame Default {
        n7 = Format Into String(format string="%s-%s", w24, w23) -> (resulting string=w22:string)  [unwired: 2 in, 1 out]
        n8 = Bundle By Name(cluster=w27, "Mapping.Channel"=w22) -> (w26:T1)
      }
      frame "" {
        # "No Mapping"
      }
    }
  }
  n9 = property class="BattPack"(reference=w9, "Accessors:MB Map"=w6) -> (reference out=w14:refnum<class "Battery Pack.lvclass">)  [unwired: 1 in, 1 out]
  n10 = call-parent "Defaults.vi"("error in (no error)"="error in (no error)", "MB Slave in"=w14) -> ("error out"=→"error out":errorcluster, "MB Slave out"=w3:refnum<class "Battery Pack.lvclass">)  [unwired: 8 in]
  n11 = property class="BattPack"(reference=w3, "Accessors:Timeout (ms)"=500 ("Module:Timeout (ms)")) -> (reference out=→"MB Slave out":refnum<class "Battery Pack.lvclass">)  [unwired: 1 in, 1 out]
